vi "Parse U64 H2T Regs.vi"(10 "FullyCustomTeeths In":T3, 11 "U64":T1[](array[typedef])) -> (2 "FullyCustomTeeths Out":T3)   [LabVIEW 2011, in "Engine Sim System Explorer.lvlib"]
uses:
  Engine Sim System Explorer.lvlib
  TypeDefs/FullyCustomRegs.ctl
  <userlib>/_FPGA Interface Advanced Tools/FPGA Bitfile Utility/TypeDefs/FIFO Channel.ctl
  <userlib>/_FPGA Interface Advanced Tools/FPGA Bitfile Utility/FPGA Bitfile Utility.lvlib
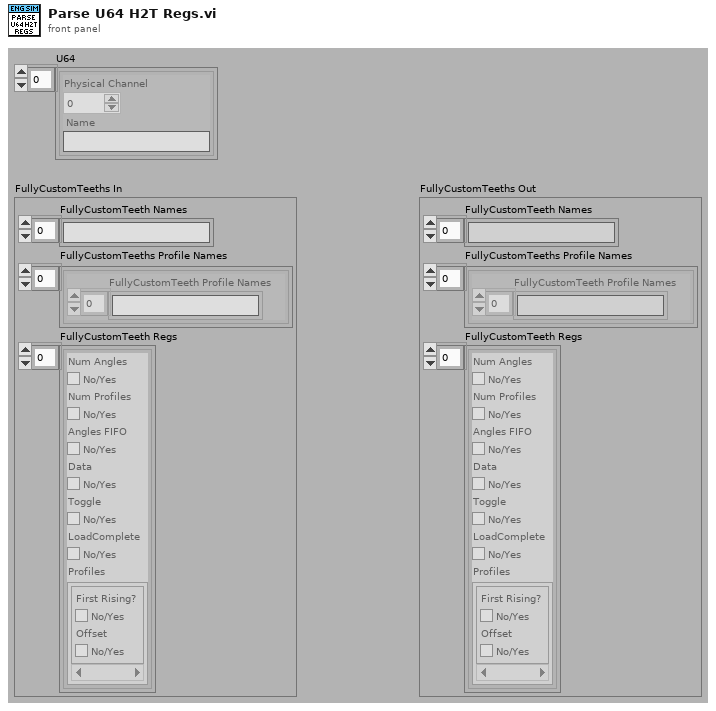
[diagram p1: front panel]
types:
  T1 = typedef "FPGA Bitfile Utility.lvlib/FIFO Channel.ctl" = cluster{"Physical Channel":u32, "Name":string}
  T2 = typedef "Engine Sim System Explorer.lvlib/FullyCustomRegs.ctl" = cluster{"Num Angles":bool, "Num Profiles":bool, "Angles FIFO":bool, "Data":bool, "Toggle":bool, "LoadComplete":bool, "Profiles":cluster{"First Rising?":bool, "Offset":bool}[]}
  T3 = cluster{"FullyCustomTeeth Names":string[], "FullyCustomTeeths Profile Names":cluster{"FullyCustomTeeth Profile Names":string[]}[], "FullyCustomTeeth Regs":T2[]}
  T4 = cluster{"FullyCustomTeeth Profile Names":string[]}
  T5 = cluster{"FullyCustomTeeth Profile Names":string[]}[]
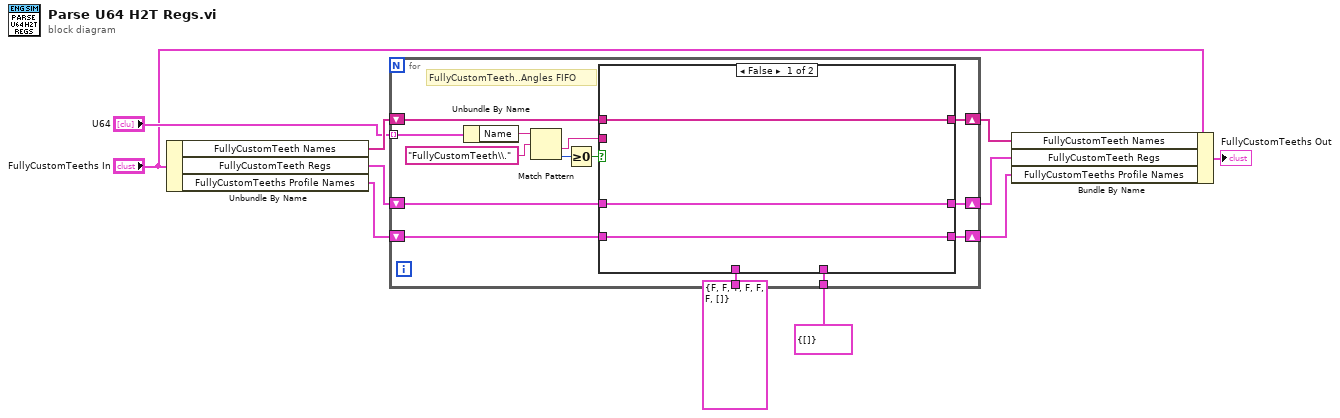
[diagram p0: block diagram]
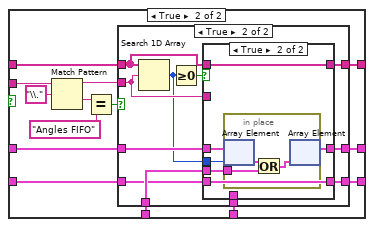
[diagram p2: hidden frame]
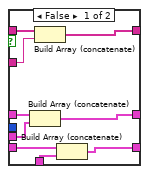
[diagram p4: hidden frame]
diagram:
  n1 = Unbundle By Name("FullyCustomTeeths In") -> ("FullyCustomTeeth Names"=w8:string[], "FullyCustomTeeth Regs"=w7:T2[], "FullyCustomTeeths Profile Names"=w3:T5)
  n2 = for {
    tunnel: "U64" -> [w25] mode=indexing
    tunnel: T2 {"Num Angles"=FALSE, "Num Profiles"=FALSE, "Angles FIFO"=TRUE, "Data"=FALSE, "Toggle"=FALSE, "LoadComplete"=FALSE, "Profiles"=[]} ("FullyCustom Registers") -> [w19]
    shift-right: [w18] -> w10
    shift-left: w7 -> [w17]
    shift-right: [w16] -> w9
    shift-left: w8 -> [w15]
    shift-right: [w12] -> w1
    shift-left: w3 -> [w14]
    tunnel: T4 {"FullyCustomTeeth Profile Names"=[]} ("FullyCustomTeeth") -> [w13]
    # "FullyCustomTeeth..Angles FIFO"
    n3 = Unbundle By Name(w25) -> ("Name"=w24:string)
    n4 = Match Pattern(string=w24, regular expression="FullyCustomTeeth\\.") -> (after substring=w20:string, offset past match=w22:i32)  [unwired: 1 in, 2 out]
    n5 = Greater Or Equal To 0?(x=w22) -> (x >= 0?=w21:bool)
    n6 = case shown="False" w21 {
      tunnel: w20 -> [_ w42]
      tunnel: w19 -> [_ w34]
      tunnel: [w27 w37] -> w18
      tunnel: w17 -> [w27 w35]
      tunnel: [w28 w38] -> w16
      tunnel: w15 -> [w28 w36]
      tunnel: w14 -> [w26 w31]
      tunnel: w13 -> [_ w30]
      tunnel: [w26 w29] -> w12
      frame False {
      }
      frame True {
        n7 = Match Pattern(string=w42, regular expression="\\.") -> (before substring=w33:string, after substring=w40:string)  [unwired: 1 in, 2 out]
        n8 = Equal?(x=w40, y="Angles FIFO") -> (x = y?=w32:bool)
        n9 = case shown="True" w32 {
          tunnel: w33 -> [_ w51]
          tunnel: w34 -> [_ w54]
          tunnel: [w44 w53] -> w37
          tunnel: w35 -> [w44 w55]
          tunnel: [w45 w50] -> w38
          tunnel: w36 -> [w45 w52]
          tunnel: w31 -> [w43 w48]
          tunnel: w30 -> [_ w47]
          tunnel: [w43 w46] -> w29
          frame False {
          }
          frame True {
            n10 = Search 1D Array(1D array=w52, element=w51) -> (index of element=w49:i32)  [unwired: 1 in]
            n11 = Greater Or Equal To 0?(x=w49) -> (x >= 0?=w56:bool)
            n12 = case shown="True" w56 {
              tunnel: w55 -> [w65 w70]
              tunnel: w54 -> [w64 w68]
              tunnel: [w63 w67] -> w53
              tunnel: w52 -> [w62 w71]
              tunnel: w51 -> [w61 _]
              tunnel: [w60 w71] -> w50
              tunnel: w49 -> [_ w69]
              tunnel: w48 -> [w59 w66]
              tunnel: w47 -> [w58 _]
              tunnel: [w57 w66] -> w46
              frame False {
                n13 = Build Array (concatenate)(w65, w64) -> (w63:T2[])
                n14 = Build Array (concatenate)(w62, w61) -> (w60:string[])
                n15 = Build Array (concatenate)(w59, w58) -> (w57:T5)
              }
              frame True {
                n16 = in-place {
                  in-place-border: w68 -> [w73]
                  n17 = in-place-array #1(w70, w69) -> (w74:T2)
                  n18 = Or(x=w74, y=w73) -> (x .or. y?=w72:T2)
                  n19 = in-place-array #1(w72) -> (w67:T2[])  [unwired: 1 out]
                }
              }
            }
          }
        }
      }
    }
  }
  n20 = Bundle By Name(cluster="FullyCustomTeeths In", "FullyCustomTeeth Names"=w9, "FullyCustomTeeth Regs"=w10, "FullyCustomTeeths Profile Names"=w1) -> (→"FullyCustomTeeths Out":T3)
